vi "CRYDV MARK LIB.vi"(0 "sAction":string="asada", 1 "DataView Array Index":i32, 2 "Docking_Update":bool=TRUE, 3 "MousePos":T2) -> (9 "Rect_Out":T1, 10 "bResult":bool=TRUE)   [LabVIEW 2013]
uses:
  <vilib>/Utility/miscctls.llb/LVRectTypeDef.ctl
  CRYNew View Global.vi
panel:
  in  "Rect_SUB":T1[](array[typedef])
  in  "Rect_LRAB":T1[](array[typedef])
  in  "Rect_Main":T1
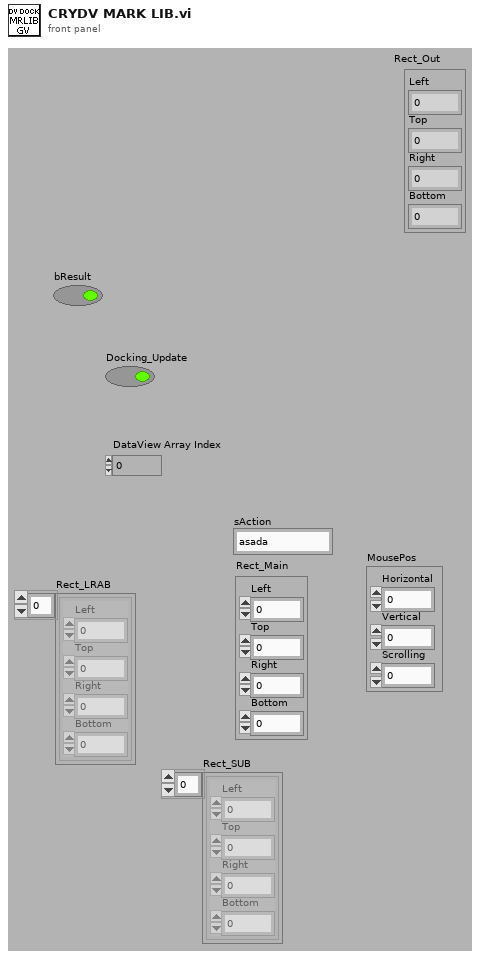
[diagram p1: front panel]
types:
  T1 = typedef "LVRectTypeDef.ctl" = cluster{"Left":i16, "Top":i16, "Right":i16, "Bottom":i16}
  T2 = cluster{"Horizontal":i32, "Vertical":i32, "Scrolling":i32}
  T3 = typedef "Graph Main Info Cluster.ctl" = cluster{"Selected_BarIdx":i32, "Selected_PanelIdx":i32, "Graph Main VIRef":refnum<vi>, "ToolBarClick":bool, "Spliter Ref Array":refnum<vi>[], "Panel Ref Array":refnum<vi>[], "Spliter_matrix":i32[][], "Panel_matrix":i32[][], "child_spliterIdx_matrix":i32[][], "split_pos_matrix":i32[][], "Title State":bool, "sQueueName":string, "Frame nID":i32, "Graph VIRef Array":cluster{"Graph VIRef":refnum<vi>, "Panel Idx":i32, "Frame VIRef":refnum<vi>, "Icon Ring":i32, "Graph Type":string}[], "View Type":string}
  T4 = enum32{"Invalid", "Standard", "Closed", "Hidden", "Minimized", "Maximized"}
  T5 = enum32{"Invalid", "Default", "Floating", "Floating/Auto-Hide", "Modal"}
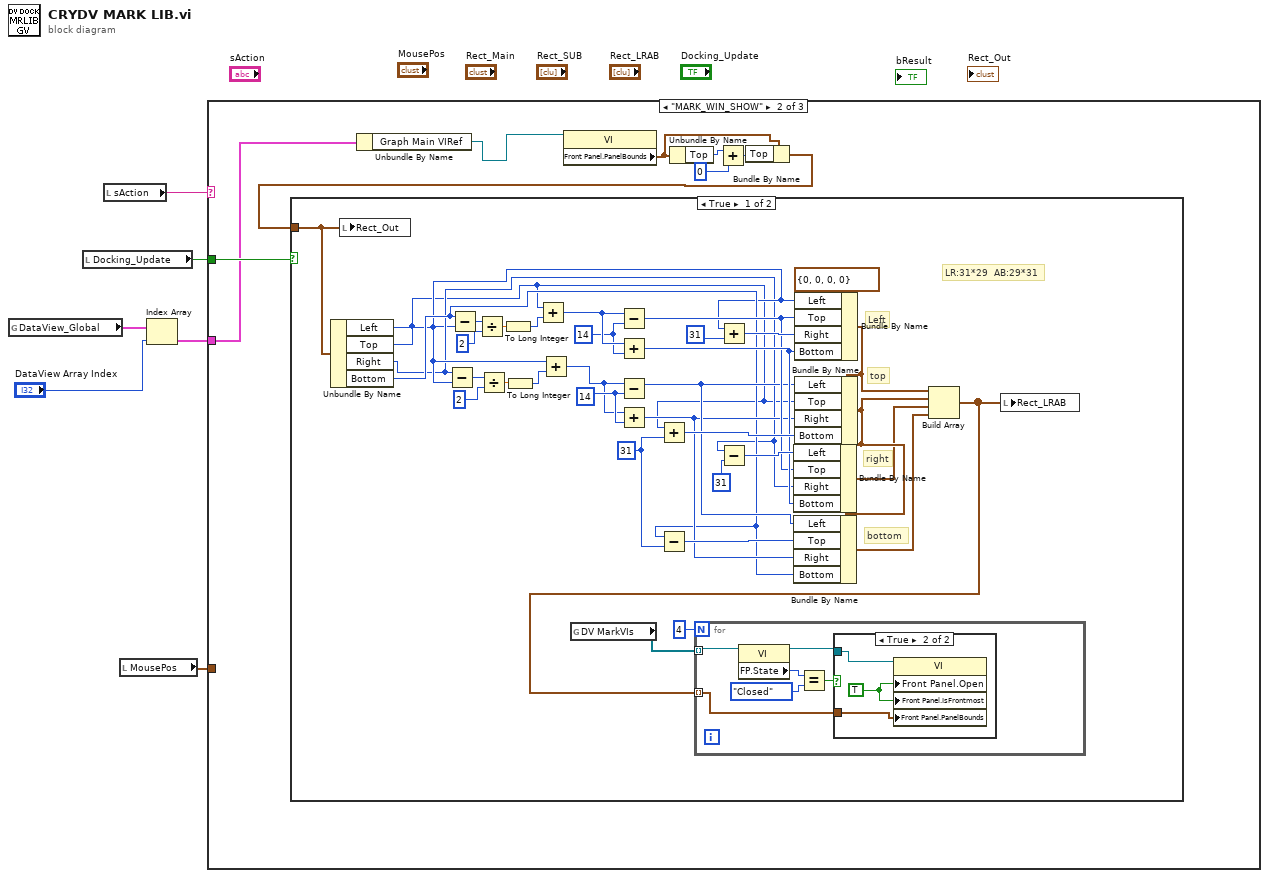
[diagram p0: block diagram]
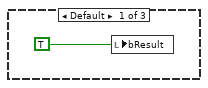
[diagram p2: hidden frame]
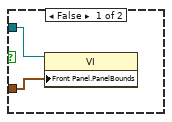
[diagram p3: hidden frame]
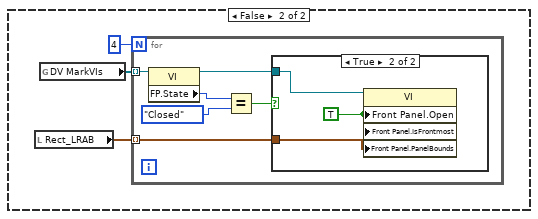
[diagram p4: hidden frame]
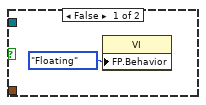
[diagram p5: hidden frame]
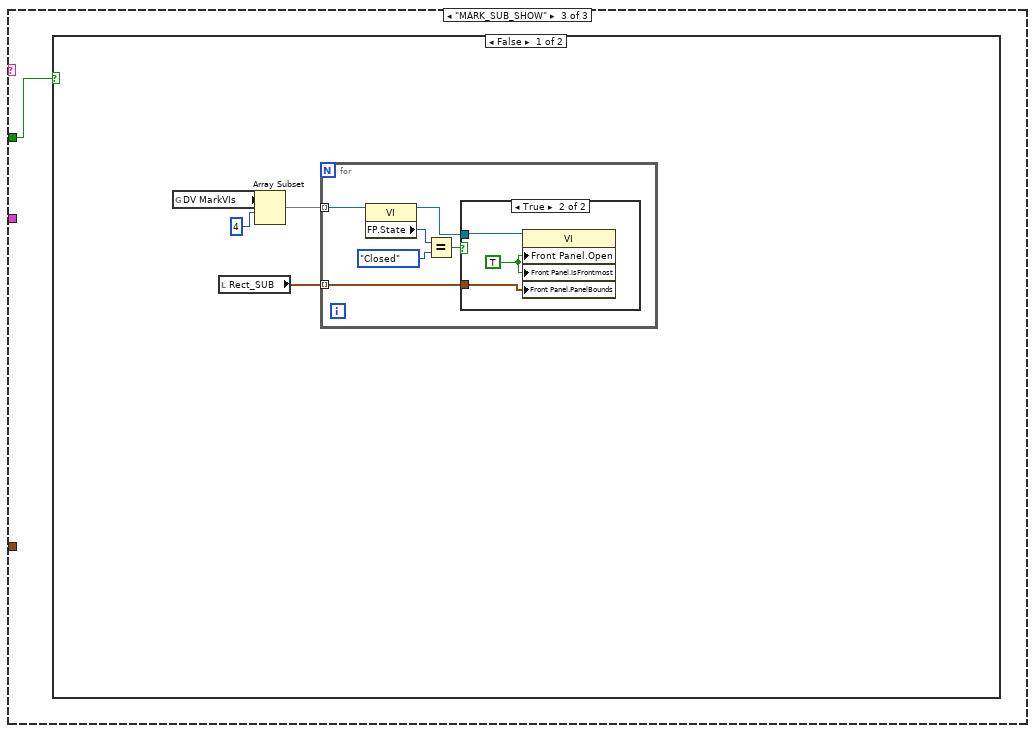
[diagram p6: hidden frame]
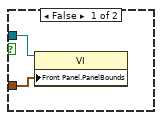
[diagram p7: hidden frame]
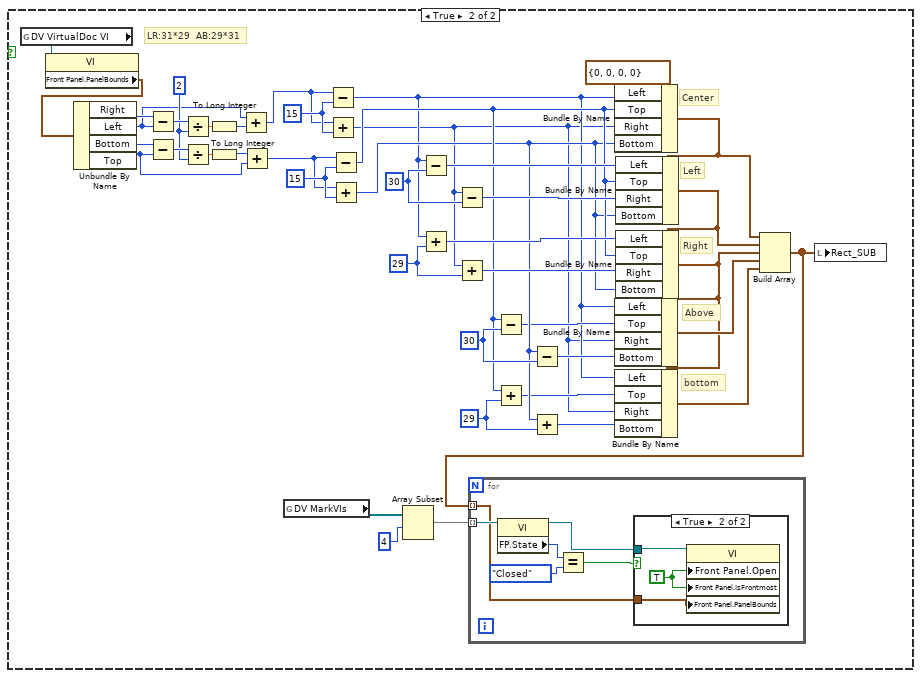
[diagram p8: hidden frame]
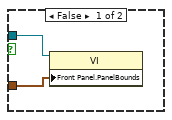
[diagram p9: hidden frame]
diagram:
  n1 = global read "CRYNew View Global.vi" "DataView_Global"() -> (w1:T3[])
  n2 = local read "Docking_Update"() -> (w4:bool)
  n3 = local read "sAction"() -> (w6:string)
  n4 = local read "MousePos"() -> (w5:T2)
  n5 = Index Array(array=w1, index="DataView Array Index") -> (element=w2:T3)
  n6 = case shown="\"MARK_WIN_SHOW\"" w6 {
    tunnel: w5 -> [_ _ _]
    tunnel: w4 -> [_ w15 w76]
    tunnel: w2 -> [_ w8 _]
    frame Default {
      n7 = local write "bResult"(TRUE ("bResult")) -> ()
    }
    frame "MARK_WIN_SHOW" {
      n8 = Unbundle By Name(w8) -> ("Graph Main VIRef"=w14:refnum<vi>)
      n9 = property class="VI"(reference=w14) -> ("Front Panel.PanelBounds"=w13:T1)  [unwired: 1 in, 2 out]
      n10 = Unbundle By Name(w13) -> ("Top"=w12:i16)
      n11 = Add(x=w12, y=i16 0) -> (x+y=w10:i16)
      n12 = Bundle By Name(cluster=w13, "Top"=w10) -> (w9:T1)
      n13 = case shown="True" w15 {
        tunnel: w9 -> [w16 _]
        frame True {
          w33 = 14
          w40 = 31
          w36 = 14
          # "LR:31*29  AB:29*31"
          # "bottom"
          # "right"
          # "top"
          # "Left"
          n14 = Unbundle By Name(w16) -> ("Left"=w25:i16, "Top"=w21:i16, "Right"=w24:i16, "Bottom"=w28:i16)
          n15 = local write "Rect_Out"(w16) -> ()
          n16 = Subtract(x=w24, y=w25) -> (x-y=w43:i16)
          n17 = Subtract(x=w28, y=w21) -> (x-y=w20:i16)
          n18 = Divide(x=w20, y=2) -> (x/y=w18:dbl)
          n19 = Divide(x=w43, y=2) -> (x/y=w23:dbl)
          n20 = To Long Integer(number=w18) -> (32bit integer=w17:i32)
          n21 = To Long Integer(number=w23) -> (32bit integer=w22:i32)
          n22 = Add(x=w21, y=w17) -> (x+y=w37:i32)
          n23 = Add(x=w25, y=w22) -> (x+y=w32:i32)
          n24 = global read "CRYNew View Global.vi" "DV MarkVIs"() -> (w47:refnum<vi>[])
          n25 = Subtract(x=w37, y=w36) -> (x-y=w34:i32)
          n26 = Add(x=w37, y=w36) -> (x+y=w35:i32)
          n27 = Subtract(x=w32, y=w33) -> (x-y=w31:i32)
          n28 = Add(x=w32, y=w33) -> (x+y=w30:i32)
          n29 = Add(x=w21, y=w40) -> (x+y=w41:i32)
          n30 = Subtract(x=w28, y=w40) -> (x-y=w39:i32)
          n31 = Add(x=w25, y=31) -> (x+y=w38:i32)
          n32 = Subtract(x=w24, y=31) -> (x-y=w42:i32)
          n33 = Bundle By Name(cluster=T1 {"Left"=0, "Top"=0, "Right"=0, "Bottom"=0} ("Front Panel Window:Panel Bounds"), "Left"=w25, "Top"=w34, "Right"=w38, "Bottom"=w35) -> (w51:T1)
          n34 = Bundle By Name(cluster=w51, "Left"=w31, "Top"=w21, "Right"=w30, "Bottom"=w41) -> (w50:T1)
          n35 = Bundle By Name(cluster=w50, "Left"=w42, "Top"=w34, "Right"=w24, "Bottom"=w35) -> (w49:T1)
          n36 = Bundle By Name(cluster=w50, "Left"=w31, "Top"=w39, "Right"=w30, "Bottom"=w28) -> (w48:T1)
          n37 = Build Array(w51, w50, w49, w48) -> (w19:T1[])
          n38 = for {
            N: 4 -> [_]
            tunnel: w19 -> [w52] mode=indexing
            tunnel: w47 -> [w57] mode=indexing
            n39 = property class="VI"(reference=w57) -> (reference out=w56:refnum<vi>, "FP.State"=w55:T4)  [unwired: 1 in, 1 out]
            n40 = Equal?(x=w55, y=T4."Closed" ("Front Panel Window:State")) -> (x = y?=w53:bool)
            n41 = case shown="True" w53 {
              tunnel: w56 -> [w59 w60]
              tunnel: w52 -> [w58 w62]
              frame False {
                n42 = property class="VI"(reference=w59, "Front Panel.PanelBounds"=w58) -> ()  [unwired: 1 in, 2 out]
              }
              frame True {
                w61 = TRUE ("Front Panel Window:Open")
                n43 = property class="VI"(reference=w60, "Front Panel.Open"=w61, "Front Panel.IsFrontmost"=w61, "Front Panel.PanelBounds"=w62) -> ()  [unwired: 1 in, 2 out]
              }
            }
          }
          n44 = local write "Rect_LRAB"(w19) -> ()
        }
        frame False {
          n45 = local read "Rect_LRAB"() -> (w63:T1[])
          n46 = global read "CRYNew View Global.vi" "DV MarkVIs"() -> (w65:refnum<vi>[])
          n47 = for {
            N: 4 -> [_]
            tunnel: w65 -> [w68] mode=indexing
            tunnel: w63 -> [w66] mode=indexing
            n48 = property class="VI"(reference=w68) -> (reference out=w67:refnum<vi>, "FP.State"=w71:T4)  [unwired: 1 in, 1 out]
            n49 = Equal?(x=w71, y=T4."Closed" ("Front Panel Window:State")) -> (x = y?=w69:bool)
            n50 = case shown="True" w69 {
              tunnel: w67 -> [_ w75]
              tunnel: w66 -> [_ w73]
              frame False {
                n51 = property class="VI"("FP.Behavior"=T5."Floating" ("Front Panel Window:Behavior")) -> ()  [unwired: 2 in, 2 out]
              }
              frame True {
                w74 = TRUE ("Front Panel Window:Open")
                n52 = property class="VI"(reference=w75, "Front Panel.Open"=w74, "Front Panel.IsFrontmost"=w74, "Front Panel.PanelBounds"=w73) -> ()  [unwired: 1 in, 2 out]
              }
            }
          }
        }
      }
    }
    frame "MARK_SUB_SHOW" {
      n53 = case shown="False" w76 {
        frame False {
          n54 = global read "CRYNew View Global.vi" "DV MarkVIs"() -> (w79:refnum<vi>[])
          n55 = local read "Rect_SUB"() -> (w77:T1[])
          n56 = Array Subset(array=w79, index=4) -> (w80:refnum<vi>[])  [unwired: 1 in]
          n57 = for {
            tunnel: w80 -> [w82] mode=indexing
            tunnel: w77 -> [w81] mode=indexing
            n58 = property class="VI"(reference=w82) -> (reference out=w83:refnum<vi>, "FP.State"=w84:T4)  [unwired: 1 in, 1 out]
            n59 = Equal?(x=w84, y=T4."Closed" ("Front Panel Window:State")) -> (x = y?=w86:bool)
            n60 = case shown="True" w86 {
              tunnel: w83 -> [w88 w90]
              tunnel: w81 -> [w87 w89]
              frame False {
                n61 = property class="VI"(reference=w88, "Front Panel.PanelBounds"=w87) -> ()  [unwired: 1 in, 2 out]
              }
              frame True {
                w91 = TRUE ("Front Panel Window:Open")
                n62 = property class="VI"(reference=w90, "Front Panel.Open"=w91, "Front Panel.IsFrontmost"=w91, "Front Panel.PanelBounds"=w89) -> ()  [unwired: 1 in, 2 out]
              }
            }
          }
        }
        frame True {
          w93 = 29
          w94 = 29
          w106 = 30
          w118 = 15
          w109 = 30
          w132 = 15
          w121 = 2
          # "Center"
          # "LR:31*29  AB:29*31"
          # "bottom"
          # "Above"
          # "Right"
          # "Left"
          n63 = global read "CRYNew View Global.vi" "DV VirtualDoc VI"() -> (w92:refnum<vi>)
          n64 = property class="VI"(reference=w92) -> ("Front Panel.PanelBounds"=w127:T1)  [unwired: 1 in, 2 out]
          n65 = Unbundle By Name(w127) -> ("Right"=w126:i16, "Left"=w116:i16, "Bottom"=w124:i16, "Top"=w115:i16)
          n66 = Subtract(x=w126, y=w116) -> (x-y=w125:i16)
          n67 = Subtract(x=w124, y=w115) -> (x-y=w122:i16)
          n68 = Divide(x=w125, y=w121) -> (x/y=w133:dbl)
          n69 = Divide(x=w122, y=w121) -> (x/y=w123:dbl)
          n70 = To Long Integer(number=w133) -> (32bit integer=w117:i32)
          n71 = To Long Integer(number=w123) -> (32bit integer=w114:i32)
          n72 = Add(x=w116, y=w117) -> (x+y=w113:i32)
          n73 = Add(x=w114, y=w115) -> (x+y=w112:i32)
          n74 = global read "CRYNew View Global.vi" "DV MarkVIs"() -> (w97:refnum<vi>[])
          n75 = Subtract(x=w113, y=w118) -> (x-y=w99:i32)
          n76 = Add(x=w113, y=w118) -> (x+y=w98:i32)
          n77 = Subtract(x=w112, y=w132) -> (x-y=w105:i32)
          n78 = Add(x=w112, y=w132) -> (x+y=w104:i32)
          n79 = Array Subset(array=w97, index=4) -> (w96:refnum<vi>[])  [unwired: 1 in]
          n80 = Subtract(x=w99, y=w109) -> (x-y=w111:i32)
          n81 = Add(x=w99, y=w94) -> (x+y=w108:i32)
          n82 = Subtract(x=w98, y=w109) -> (x-y=w110:i32)
          n83 = Add(x=w98, y=w94) -> (x+y=w107:i32)
          n84 = Subtract(x=w105, y=w106) -> (x-y=w103:i32)
          n85 = Add(x=w105, y=w93) -> (x+y=w101:i32)
          n86 = Subtract(x=w104, y=w106) -> (x-y=w102:i32)
          n87 = Add(x=w104, y=w93) -> (x+y=w100:i32)
          n88 = Bundle By Name(cluster=T1 {"Left"=0, "Top"=0, "Right"=0, "Bottom"=0} ("Front Panel Window:Panel Bounds"), "Left"=w99, "Top"=w105, "Right"=w98, "Bottom"=w104) -> (w119:T1)
          n89 = Bundle By Name(cluster=w119, "Left"=w111, "Top"=w105, "Right"=w110, "Bottom"=w104) -> (w128:T1)
          n90 = Bundle By Name(cluster=w128, "Left"=w108, "Top"=w105, "Right"=w107, "Bottom"=w104) -> (w129:T1)
          n91 = Bundle By Name(cluster=w129, "Left"=w99, "Top"=w103, "Right"=w98, "Bottom"=w102) -> (w130:T1)
          n92 = Bundle By Name(cluster=w129, "Left"=w99, "Top"=w101, "Right"=w98, "Bottom"=w100) -> (w131:T1)
          n93 = Build Array(w119, w128, w129, w130, w131) -> (w95:T1[])
          n94 = for {
            tunnel: w96 -> [w137] mode=indexing
            tunnel: w95 -> [w136] mode=indexing
            n95 = property class="VI"(reference=w137) -> (reference out=w138:refnum<vi>, "FP.State"=w139:T4)  [unwired: 1 in, 1 out]
            n96 = Equal?(x=w139, y=T4."Closed" ("Front Panel Window:State")) -> (x = y?=w135:bool)
            n97 = case shown="True" w135 {
              tunnel: w138 -> [w142 w144]
              tunnel: w136 -> [w141 w143]
              frame False {
                n98 = property class="VI"(reference=w142, "Front Panel.PanelBounds"=w141) -> ()  [unwired: 1 in, 2 out]
              }
              frame True {
                w145 = TRUE ("Front Panel Window:Open")
                n99 = property class="VI"(reference=w144, "Front Panel.Open"=w145, "Front Panel.IsFrontmost"=w145, "Front Panel.PanelBounds"=w143) -> ()  [unwired: 1 in, 2 out]
              }
            }
          }
          n100 = local write "Rect_SUB"(w95) -> ()
        }
      }
    }
  }
